vi "Set Or Get NumRows.vi"(8 "error in (no error)":errorcluster caption="错误输入（无错误）", 9 "Mode":T1, 10 "NumRows In":u32, 11 "Table Ref In":refnum<vi>) -> (0 "error out":errorcluster caption="错误输出", 2 "NumRows Out":u32, 3 "Table Ref Out":refnum<vi>)   [LabVIEW 2012, in "Table Tool.lvlib"]
uses:
  Table Tool.lvlib
  GetOrSet.ctl
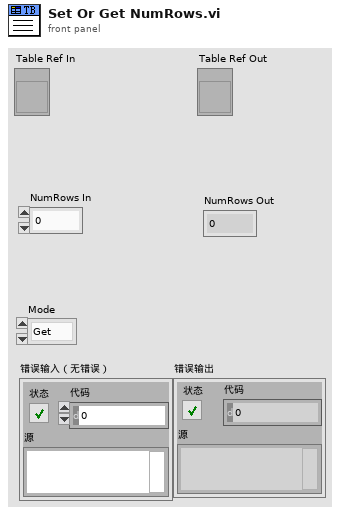
[diagram p1: front panel]
types:
  T1 = typedef "Table Tool.lvlib/GetOrSet.ctl" = enum16{"Get", "Set"}
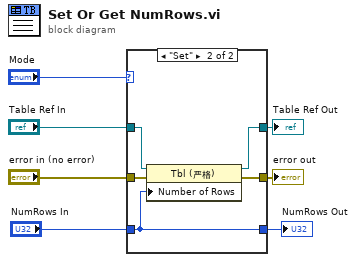
[diagram p0: block diagram]
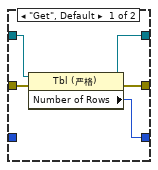
[diagram p2: hidden frame]
diagram:
  n1 = case shown="\"Set\"" "Mode" {
    tunnel: "Table Ref In" -> [w11 w16]
    tunnel: "error in (no error)" -> [w12 w17]
    tunnel: [w9 w14] -> w4
    tunnel: [w10 w15] -> w3
    tunnel: [w8 w13] -> w2
    tunnel: "NumRows In" -> [_ w13]
    frame "Get", Default {
      n2 = property class="Tbl (严格)"(reference=w11, error in=w12) -> (reference out=w10:refnum<vi>, error out=w9:errorcluster, "Number of Rows"=w8:u32)
    }
    frame "Set" {
      n3 = property class="Tbl (严格)"(reference=w16, error in=w17, "Number of Rows"=w13) -> (reference out=w15:refnum<vi>, error out=w14:errorcluster)
    }
  }
  "Table Ref Out" <- w3
  "error out" <- w4
  "NumRows Out" <- w2
